vi "Pixel to Global Position.vi"(7 "picture info":T1={"picture size"={"Width"=500, "Height"=500}, "pixels per unit"=10.0}, 10 "pixel y":i32, 11 "pixel x":i32) -> (2 "global y":dbl, 3 "global x":dbl)   [LabVIEW 2017, in "NI_Robotics_Steering Picture.lvlib"]
uses:
  <vilib>/robotics/Utilities/Visualization/Steering Visualization/Steering Picture/NI_Robotics_Steering Picture.lvlib
  <vilib>/robotics/Utilities/Visualization/Steering Visualization/Steering Picture/Picture Info.ctl
  <vilib>/Utility/miscctls.llb/LVBoundsTypeDef.ctl
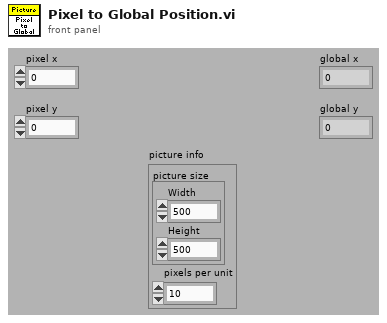
[diagram p1: front panel]
types:
  T1 = typedef "NI_Robotics_Steering Picture.lvlib/Picture Info.ctl" = cluster{"picture size":T2, "pixels per unit":dbl}
  T2 = typedef "LVBoundsTypeDef.ctl" = cluster{"Width":u32, "Height":u32}
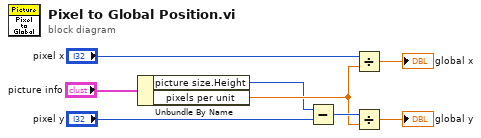
[diagram p0: block diagram]
diagram:
  n1 = Unbundle By Name("picture info") -> ("picture size.Height"=w1:u32, "pixels per unit"=w2:dbl)
  n2 = Subtract(x=w1, y="pixel y") -> (x-y=w5:u32)
  n3 = Divide(x="pixel x", y=w2) -> (x/y=→"global x":dbl)
  n4 = Divide(x=w5, y=w2) -> (x/y=→"global y":dbl)
